vi "Get Reference.vi"(8 "error in (no error)":errorcluster, 10 "Samples":i32, 11 "Lock-in Detector in":refnum<class "Lock-in Detector.lvclass">) -> (0 "error out":errorcluster, 2 "Reference":cdb[](array[numeric]), 3 "Lock-in Detector out":refnum<class "Lock-in Detector.lvclass">)   [LabVIEW 2020, in "Lock-in Detector.lvclass"]
uses:
  Lock-in Detector.lvclass
  Lock-in Detector.lvclass/Lock-in Detector.ctl
  Write Reference phase.vi
  Read Reference amplitude.vi
  Read Reference frequency.vi
  Read Harmonic.vi
  Read Reference phase.vi
  <vilib>/Analysis/NI_AALBase.lvlib
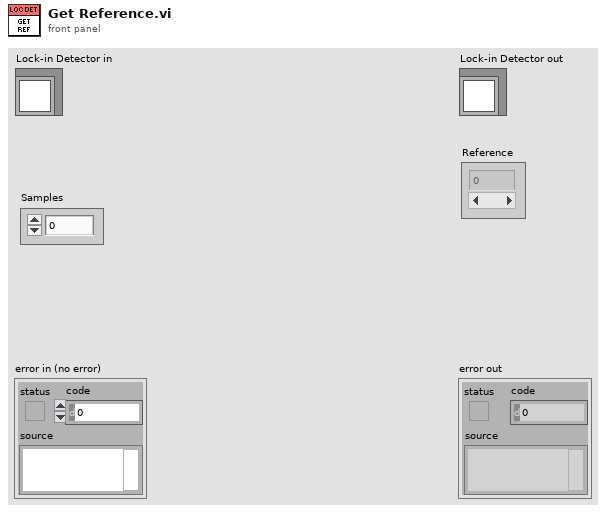
[diagram p1: front panel]
types:
  T1 = typedef "Lockin Parameters.ctl" = cluster{"Frequency":dbl, "Phase":dbl, "Syncronous":bool, "Points per sine wave":i32, "DDS":bool, "Frequency word":u32, "Phase word":u32, "DDS modulus":i64, "DDS clock":dbl}
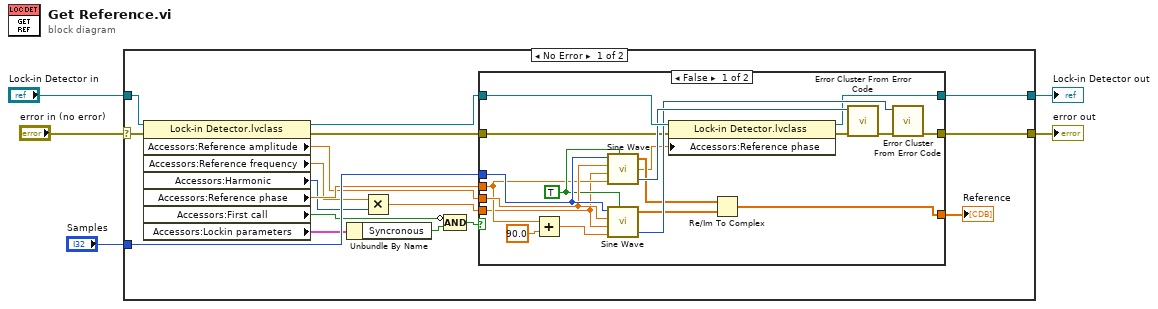
[diagram p0: block diagram]
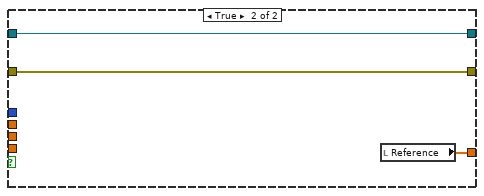
[diagram p2: hidden frame]
diagram:
  n1 = case shown="No Error" "error in (no error)" {
    selector: "error in (no error)" -> [w21 w46]
    tunnel: [w20 w46] -> w4
    tunnel: [w19 w45] -> w2
    tunnel: "Lock-in Detector in" -> [w14 w45]
    tunnel: "Samples" -> [w22 _]
    frame No Error {
      n2 = property class="Lock-in Detector.lvclass"(reference=w14, error in=w21) -> (reference out=w13:refnum<class "Lock-in Detector.lvclass">, error out=w15:errorcluster, "Accessors:Reference amplitude"=w6:dbl, "Accessors:Reference frequency"=w7:dbl, "Accessors:Harmonic"=w8:i32, "Accessors:Reference phase"=w9:dbl, "Accessors:First call"=w11:bool, "Accessors:Lockin parameters"=w12:T1)
      n3 = Unbundle By Name(w12) -> ("Syncronous"=w10:bool)
      n4 = Multiply(x=w7, y=w8) -> (x*y=w16:dbl)
      n5 = Compound Arithmetic op=AND(invert w11, w10) -> (w17:bool)
      n6 = case shown="False" w17 {
        tunnel: w22 -> [w39 _]
        tunnel: w13 -> [w38 w43]
        tunnel: w6 -> [w37 _]
        tunnel: w15 -> [w33 w42]
        tunnel: [w31 w42] -> w20
        tunnel: w9 -> [w30 _]
        tunnel: [w24 w43] -> w19
        tunnel: w16 -> [w29 _]
        tunnel: [w26 w44] -> w18
        frame False {
          w36 = TRUE ("reset phase")
          n7 = Add(x=w30, y=90.0) -> (x+y=w40:dbl)
          n8 = call <vilib>:"Sine Wave.vi"("samples"=w39, "amplitude"=w37, "frequency"=w29, "phase in"=w30, "reset phase"=w36) -> ("sine wave"=w28:dbl[], "phase out"=w23:dbl, "error"=w35:i32)
          n9 = call <vilib>:"Sine Wave.vi"("samples"=w39, "amplitude"=w37, "frequency"=w29, "phase in"=w40, "reset phase"=w36) -> ("sine wave"=w27:dbl[], "error"=w34:i32)  [unwired: 1 out]
          n10 = property class="Lock-in Detector.lvclass"(reference=w38, error in=w33, "Accessors:Reference phase"=w23) -> (reference out=w24:refnum<class "Lock-in Detector.lvclass">, error out=w25:errorcluster)
          n11 = Re/Im To Complex(1:w27, 2:w28) -> (0:w26:cdb[])
          n12 = call <vilib>:"Error Cluster From Error Code.vi"("error in (no error)"=w25, "error code (0)"=w35) -> ("error out"=w32:errorcluster)  [unwired: 7 in]
          n13 = call <vilib>:"Error Cluster From Error Code.vi"("error in (no error)"=w32, "error code (0)"=w34) -> ("error out"=w31:errorcluster)  [unwired: 7 in]
        }
        frame True {
          n14 = local read "Reference"() -> (w44:cdb[])
        }
      }
      "Reference" <- w18
    }
    frame Error {
    }
  }
  "error out" <- w4
  "Lock-in Detector out" <- w2
